vi "optimized_eod_recorder.vi"() -> ()   [LabVIEW 2014]
uses:
  Dropbox (MSU Efish Lab)/Undergraduates/Sarah_Sam/To Github/eodrecorderstates.ctl
  <vilib>/_DAQmxBase/Internals/DAQmxBase Read (Analog 2D DBL NChan NSamp).vi
  <vilib>/_DAQmxBase/Internals/DAQmxBase Timing (Sample Clock).vi
  <vilib>/_DAQmxBase/Internals/DAQmxBase Create Channel (AI-Voltage-Basic).vi
  <vilib>/Utility/miscctls.llb/LVCursorListTypeDef.ctl
  <vilib>/Utility/error.llb/DialogType.ctl
panel:
  in  "stop":bool
  in  "index (row)":i32
  out "Tab Control 3":enum32{"Page 1", "Page 2"}(tab)
  out "Waveform Graph":waveform(dbl)(graph)
  in  "Graph Time Base (sec)":dbl=1.0 format="%#_13g"
  out "Threshold":sgl
  out "Threshold 2":sgl
  out "Waveform Graph 2":waveform(dbl)(graph)
  out "Channel Name":string
  in  "Stop":bool caption="stop"
  out "Pre-Trigger Error Indicator":bool caption="Error Indicator\n(Indicates if trigger occurs before\npre-trigger samples were acquired)"
  out "# Pretrigger Samples\nAcquired":i32
  in  "RightSideControls":T1={"Open Data"=FALSE, "Capture"=FALSE, "LiveDataMode"=FALSE, "Sample Rate  (Hz)"=10000.0, "Length (Sec)"=0.05}
  out "ModeDisplay":string
  in  "Device in":tag="Dev1"
  in  "Channel":tag="Dev1/ai0"
  out "Tab Control":enum32{"Live Data", "Edit Data", "View Data"}(tab)
  in  "Tab Control 2":enum32{"Enter Data", "View Data"}(tab)
  in  "RecordDataControls":T2
  in  "Path":path
  in  "Waveform_Data_Entry":T3={"Species"="", "Comments"="", "Recording Temp °C"="", "Locality Code"="", "Specimen No."="", "Date"="", "Time"="", "Coupling"=FALSE, "Polarity 2"=FALSE, "Gain"=10000.0} {"Gain" step=1.0 scale=1.0..50000.0 scale format="%#_6e"}
  out "EodText":string[](array[string])
  out "Polarity":i32[](array[numeric])
  out "Npts":i32[](array[numeric])
  out "Srate":i32[](array[numeric])
  out "ADRange":dbl[](array[numeric])
  in  "WaveNumber":i32(slide)=1 min=0 step=1 scale=1.0..3.0 scale format="%#.0f"
  # "EOD Recorder v. 1.0"
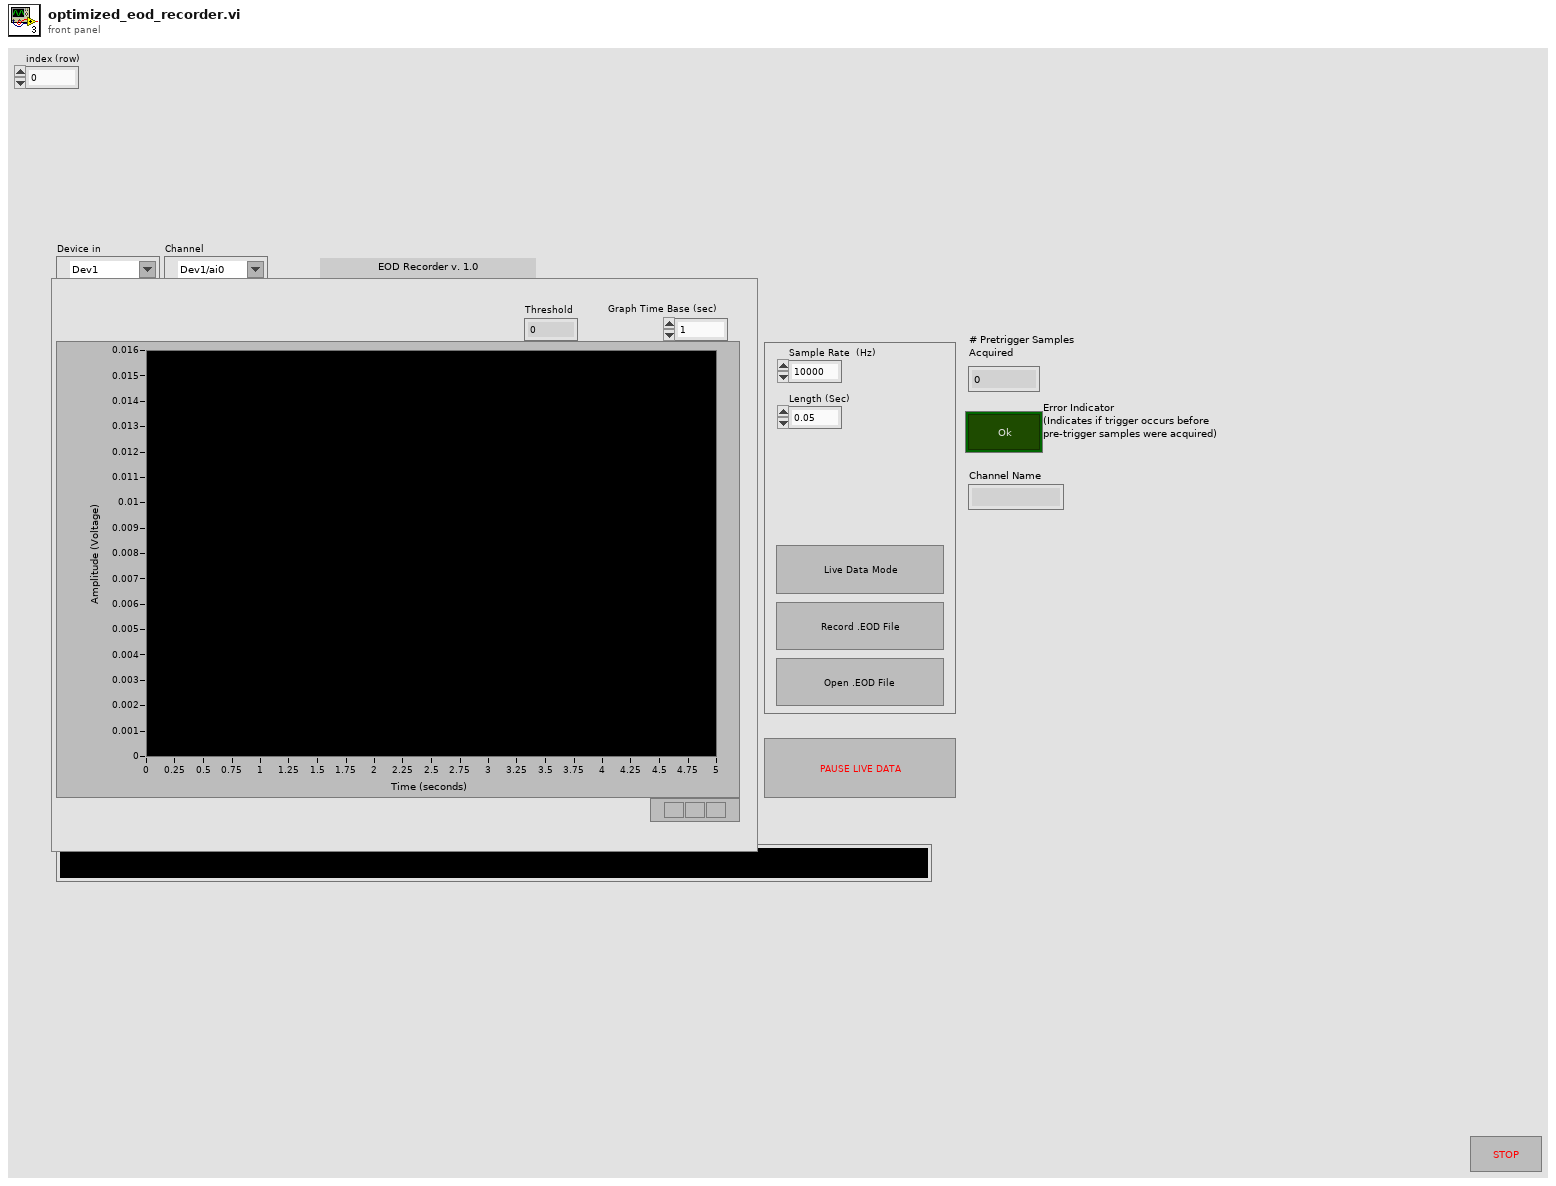
[diagram p1: front panel]
types:
  T1 = cluster{"Open Data":bool, "Capture":bool, "LiveDataMode":bool, "Sample Rate  (Hz)":dbl, "Length (Sec)":dbl}
  T2 = cluster{"Discard&Continue":bool, "Save&Finish":bool, "Save&Continue":bool, "StartOver":bool}
  T3 = cluster{"Species":string, "Comments":string, "Recording Temp °C":string, "Locality Code":string, "Specimen No.":string, "Date":string, "Time":string, "Coupling":bool, "Polarity 2":bool, "Gain":dbl}
  T4 = cluster{"Cursor.Cursor Y":dbl, "XScale.Maximum":dbl, "XScale.Minimum":dbl, "YScale.Maximum":dbl, "YScale.Minimum":dbl}
  T5 = typedef "eodrecorderstates.ctl" = enum16{"copy_scale_info", "setup", "stop", "initialize", "live data", "capture data", "analyze data", "pause live data", "open data", "display opened data", "view_collected_data", "write to file", "audio_live"}
  T6 = cluster{"data":dbl[][], "task ":refnum<k21>, "error ":errorcluster, "Min":dbl, "Max":dbl, "LastGrabbedSrate":dbl, "OpenedWaveformData":cluster{"Nchar":i32[], "EodText":string[], "Nbits":i32[], "Nbytes":i32[], "userdata":dbl[][], "Polarity":i32[], "Srate":i32[], "ADRange":dbl[], "Npts":i32[], "Wave":dbl[][]}, "NumberofWavesLoaded":i32, "lastgrabbedsamples":i32, "LastCapturedWaveformData":cluster{"Nchar":i32, "EodText":string, "Nbits":i32, "Nbytes":i32, "userdata":dbl, "Polarity":i32, "Srate":i32, "Npts":i32, "Wave":waveform(dbl), "Version":i32}}
  T7 = typedef "LVCursorListTypeDef.ctl" = cluster{"Name":string, "Color":u32, "Style":u8, "Point Style":u8, "Name Visible":bool, "Allow Drag":bool, "Cursor Mode":u32, "Plot":i32, "Index":i32, "Position":cluster{"X":dbl, "Y":dbl}, "X Scale":u32, "Y Scale":u32, "Watch Plots":i32[], "Watch All Plots":bool, "Plot Area":i32, "Label Offset":cluster{"X":dbl, "Y":dbl}}[]
  T8 = enum16{"Rising Edge", "Falling Edge", "Above Level", "Below Level", "When Inside Window", "When Outside Window"}
  T9 = enum16{"open", "replace", "create", "open or create", "replace or create", "replace or create with confirmation"}
  T10 = typedef "DialogType.ctl" = u16
  T11 = cluster{"Nchar":i32[], "EodText":string[], "Nbits":i32[], "Nbytes":i32[], "userdata":dbl[][], "Polarity":i32[], "Srate":i32[], "ADRange":dbl[], "Npts":i32[], "Wave":dbl[][]}
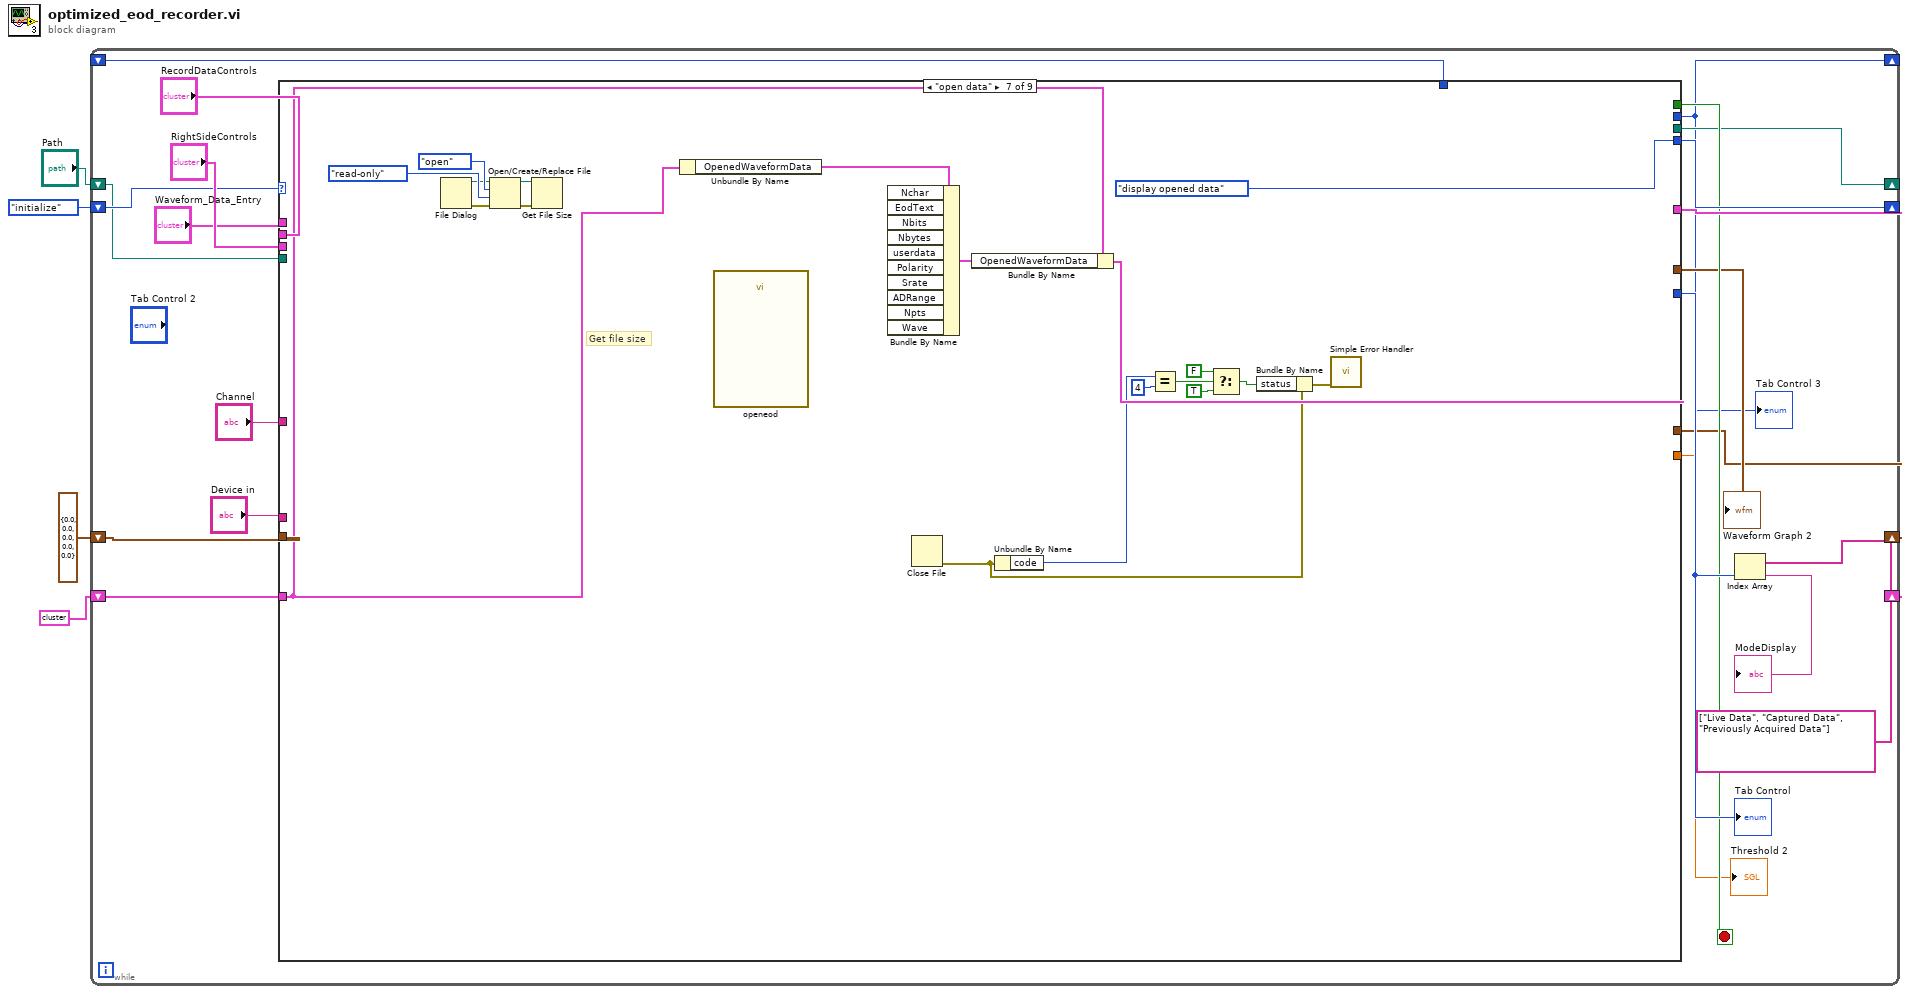
[diagram p0: block diagram]
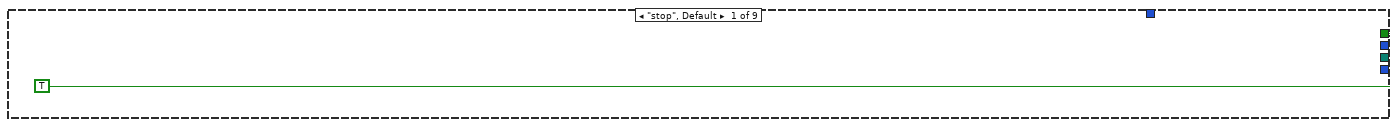
[diagram p2: hidden frame]
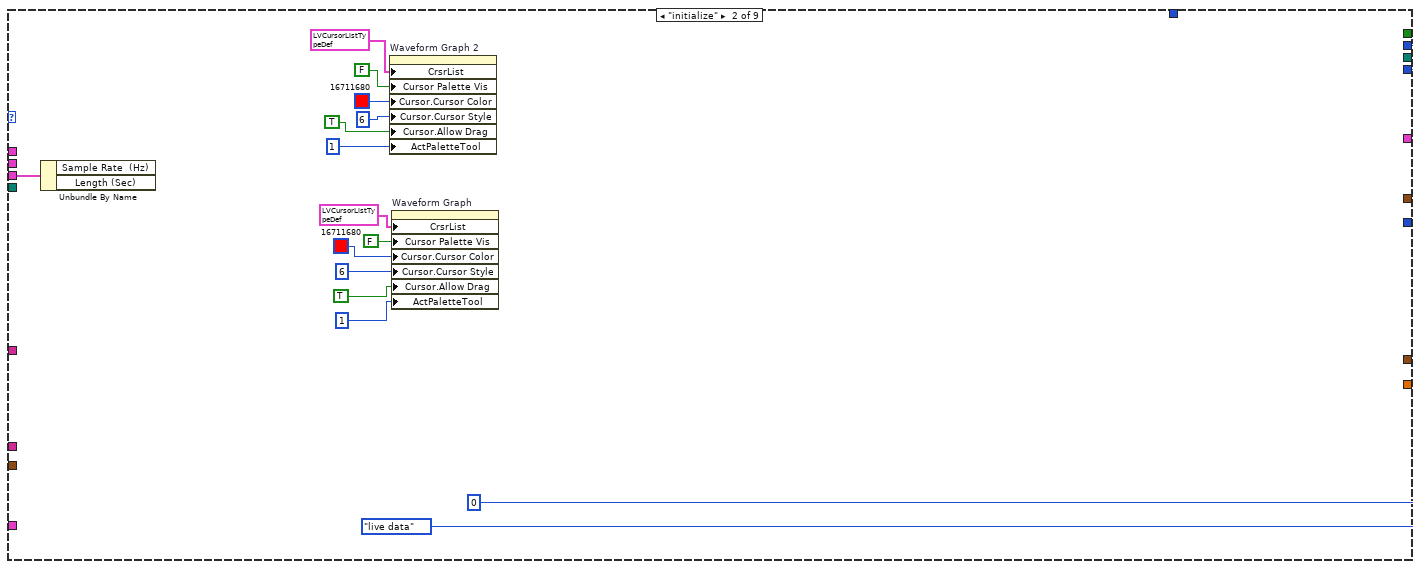
[diagram p3: hidden frame]
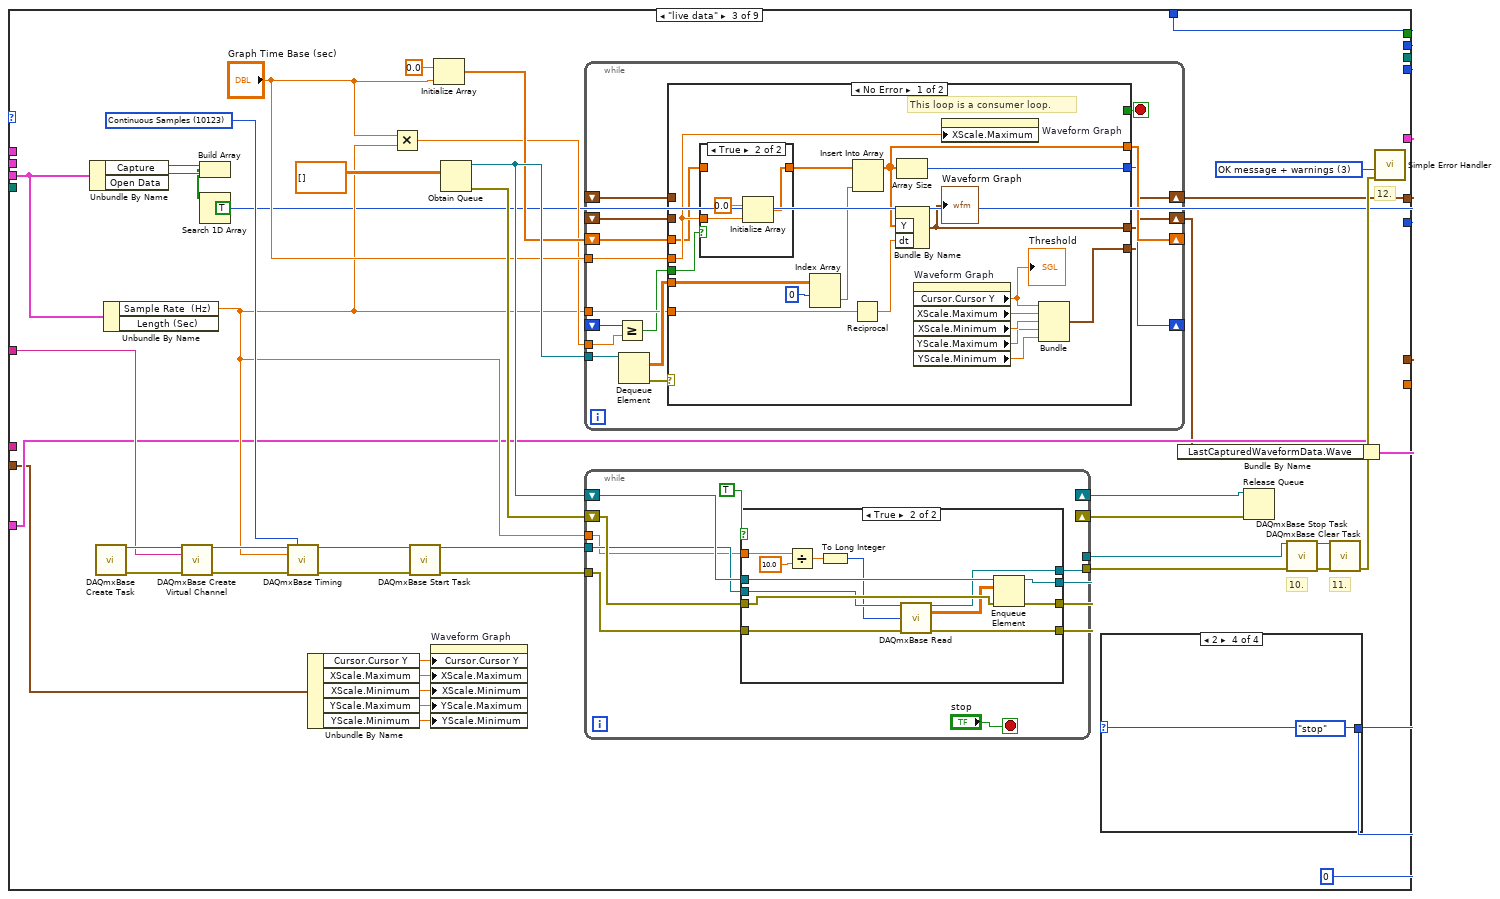
[diagram p4: hidden frame]
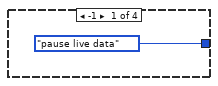
[diagram p5: hidden frame]
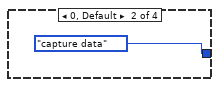
[diagram p6: hidden frame]
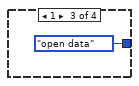
[diagram p7: hidden frame]
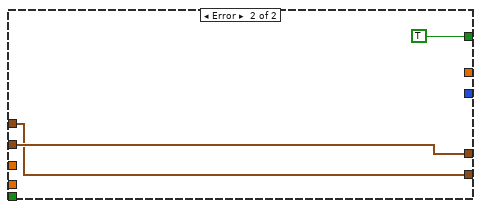
[diagram p9: hidden frame]
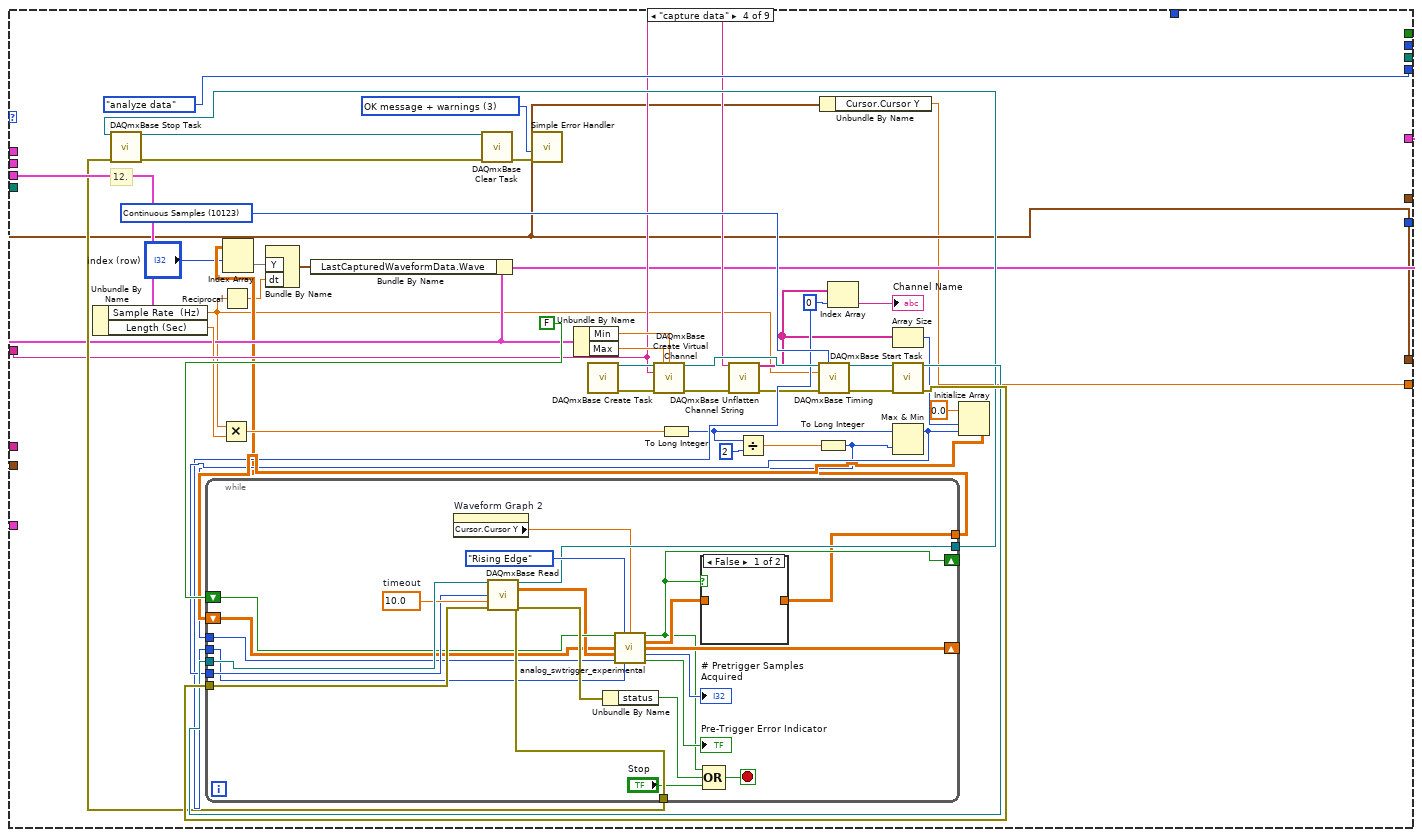
[diagram p11: hidden frame]
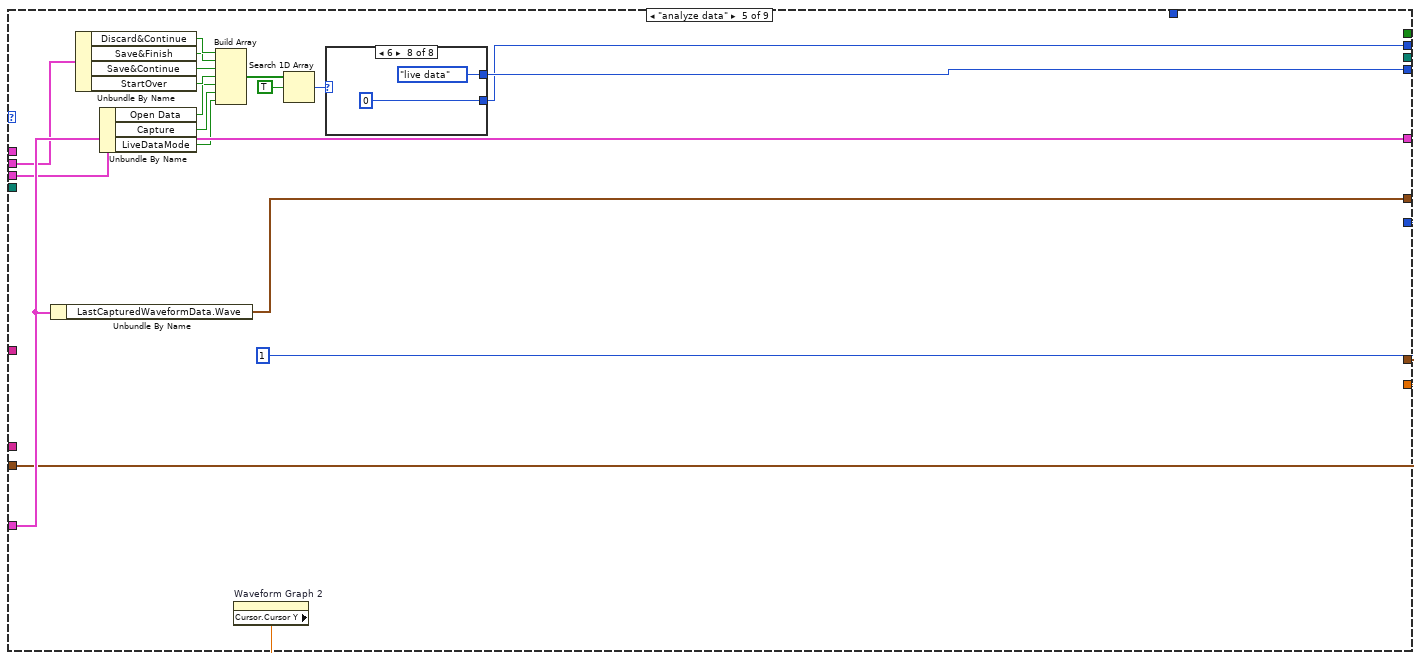
[diagram p13: hidden frame]
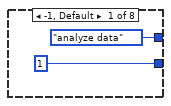
[diagram p14: hidden frame]
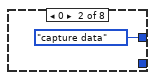
[diagram p15: hidden frame]
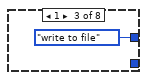
[diagram p16: hidden frame]
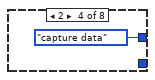
[diagram p17: hidden frame]
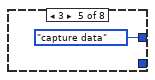
[diagram p18: hidden frame]
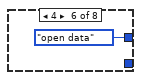
[diagram p19: hidden frame]
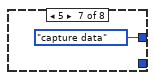
[diagram p20: hidden frame]
diagram:
  n1 = while {
    shift-right: [w21] -> _
    shift-left: T6 {"data"=[], "task "="", "error "={"status"=FALSE, "code"=0, "source"=""}, "Min"=-10.0, "Max"=10.0, "LastGrabbedSrate"=100000.0, "OpenedWaveformData"={"Nchar"=[], "EodText"=[], "Nbits"=[], "Nbytes"=[], "userdata"=[], "Polarity"=[], "Srate"=[], "ADRange"=[], "Npts"=[], "Wave"=[]}, "NumberofWavesLoaded"=4, "lastgrabbedsamples"=0, "LastCapturedWaveformData"={"Nchar"=0, "EodText"="", "Nbits"=0, "Nbytes"=0, "userdata"=0.0, "Polarity"=0, "Srate"=0, "Npts"=0, "Wave"={"t0"=timestamp(0 s since 1904-01-01), "dt"=1.0, "Y"=[]}, "Version"=0}} -> [w25]
    shift-right: [w20] -> _
    shift-left: eodrecorderstates."initialize" ("Enum") -> [w19]
    shift-right: [w12] -> _
    shift-left: "Path" -> [w13]
    shift-right: [w9] -> _
    shift-left: T4 {"Cursor.Cursor Y"=0.0, "XScale.Maximum"=0.0, "XScale.Minimum"=0.0, "YScale.Maximum"=0.0, "YScale.Minimum"=0.0} -> [w8]
    shift-right: [w6] -> _
    shift-left: _ -> [w5]
    stop <- w15 stop-if-true
    n2 = case shown="\"open data\"" w19 {
      tunnel: w25 -> [_ _ w51 w169 w246 w278 w291 w314 w343]
      tunnel: "Device in" -> [_ _ _ _ _ _ _ _ _]
      tunnel: "Channel" -> [_ _ w60 w176 _ _ _ _ _]
      tunnel: "RightSideControls" -> [_ w41 w86 w204 w234 w266 _ w305 _]
      tunnel: [_ _ w49 w168 w246 w278 w289 w314 _] -> w21
      tunnel: [_ eodrecorderstates."live data" ("Enum") w53 eodrecorderstates."analyze data" ("Enum") w237 eodrecorderstates."analyze data" ("Enum") eodrecorderstates."display opened data" ("Enum") w300 _] -> w20
      tunnel: [_ _ 0 _ 1 1 _ 2 _] -> w16
      tunnel: [TRUE _ _ _ _ _ _ _ _] -> w15
      tunnel: "Waveform_Data_Entry" -> [_ _ _ _ _ _ _ _ w351]
      tunnel: w13 -> [_ _ _ _ _ _ _ _ w337]
      tunnel: [_ _ _ _ _ _ _ _ w336] -> w12
      tunnel: "RecordDataControls" -> [_ _ _ _ w245 w277 _ _ _]
      tunnel: [_ _ _ _ w235 w267 _ _ _] -> w10
      tunnel: [_ 0 w42 _ w229 1 _ _ _] -> w6
      tunnel: [_ _ w52 w161 w228 w257 _ _ _] -> w9
      tunnel: w8 -> [_ _ w48 w161 w228 w257 _ _ _]
      tunnel: [_ _ _ w160 w230 _ _ _ _] -> w7
      tunnel: w5 -> [_ _ w42 _ _ _ _ _ _]
      frame "stop", Default {
      }
      frame "initialize" {
        n3 = Unbundle By Name(w41) -> ()  [unwired: 2 out]
        n4 = property on="Waveform Graph 2" class="WFGraph (strict)"("CrsrList"=T7 [{"Name"="Threshold\n", "Color"=0, "Style"=0, "Point Style"=0, "Name Visible"=FALSE, "Allow Drag"=TRUE, "Cursor Mode"=0, "Plot"=0, "Index"=0, "Position"={"X"=-inf, "Y"=0.0}, "X Scale"=0, "Y Scale"=0, "Watch Plots"=[], "Watch All Plots"=FALSE, "Plot Area"=0, "Label Offset"={"X"=0.0, "Y"=0.0}}] ("Cursor List"), "Cursor Palette Vis"=FALSE ("Cursor Legend Visible"), "Cursor.Cursor Color"=u32 16711680, "Cursor.Cursor Style"=u8 6, "Cursor.Allow Drag"=TRUE, "ActPaletteTool"=1 ("Palette:Active Tool")) -> ()  [unwired: 2 in, 2 out]
        n5 = property on="Waveform Graph" class="WFGraph (strict)"("CrsrList"=T7 [{"Name"="Threshold\n", "Color"=0, "Style"=0, "Point Style"=0, "Name Visible"=FALSE, "Allow Drag"=TRUE, "Cursor Mode"=0, "Plot"=0, "Index"=0, "Position"={"X"=-inf, "Y"=0.0}, "X Scale"=0, "Y Scale"=0, "Watch Plots"=[], "Watch All Plots"=FALSE, "Plot Area"=0, "Label Offset"={"X"=0.0, "Y"=0.0}}] ("Cursor List"), "Cursor Palette Vis"=FALSE ("Cursor Legend Visible"), "Cursor.Cursor Color"=u32 16711680, "Cursor.Cursor Style"=u8 6, "Cursor.Allow Drag"=TRUE, "ActPaletteTool"=1 ("Palette:Active Tool")) -> ()  [unwired: 2 in, 2 out]
      }
      frame "live data" {
        w66 = T10 3 items=["no dialog", "OK message", "continue or stop message", "OK message + warnings", "continue/stop + warnings"] ("type of dialog (OK msg:1)")
        w72 = 10123 items=["Finite Samples"=10178, "Continuous Samples"=10123, "Hardware Timed Single Point"=12522] ("sample mode")
        # "12."
        # "11."
        # "10."
        n6 = Unbundle By Name(w86) -> ("Capture"=w58:bool, "Open Data"=w57:bool)
        n7 = call <vilib>:"DAQmxBase Create Task.vi"() -> ("task out"=w80:refnum<k21>, "error out"=w79:errorcluster)  [unwired: 5 in, 9 out]
        n8 = Unbundle By Name(w86) -> ("Sample Rate  (Hz)"=w59:dbl)  [unwired: 1 out]
        n9 = call-poly <vilib>:"DAQmxBase Create Virtual Channel.vi"("task in"=w80, "physical channels"=w60, "error in"=w79) -> ("task out"=w78:refnum<k21>, "error out"=w77:errorcluster)  [unwired: 6 in, 5 out]
        n10 = Build Array(w58, w57) -> (w56:bool[])
        n11 = Search 1D Array(1D array=w56, element=TRUE) -> (index of element=w54:i32)  [unwired: 1 in]
        n12 = call-poly <vilib>:"DAQmxBase Timing.vi"("task/channels in"=w78, "sample mode"=w72, "rate"=w59, "error in"=w77) -> ("task out"=w76:refnum<k21>, "error out"=w75:errorcluster)  [unwired: 3 in, 7 out]
        n13 = Unbundle By Name(w48) -> ("Cursor.Cursor Y"=w47:dbl, "XScale.Maximum"=w46:dbl, "XScale.Minimum"=w45:dbl, "YScale.Maximum"=w44:dbl, "YScale.Minimum"=w43:dbl)
        n14 = Multiply(x="Graph Time Base (sec)", y=w59) -> (x*y=w61:dbl)
        n15 = call <vilib>:"DAQmxBase Start Task.vi"("task/channels in"=w76, "error in"=w75) -> ("task out"=w74:refnum<k21>, "error out"=w73:errorcluster)  [unwired: 12 out]
        n16 = property on="Waveform Graph" class="WFGraph (strict)"("Cursor.Cursor Y"=w47, "XScale.Maximum"=w46, "XScale.Minimum"=w45, "YScale.Maximum"=w44, "YScale.Minimum"=w43) -> ()  [unwired: 2 in, 2 out]
        n17 = Initialize Array(0.0 ("element"), "Graph Time Base (sec)") -> (w63:dbl[])
        n18 = Obtain Queue(element data type=dbl[][] [] ("data")) -> (queue out=w84:refnum<queue>, error out=w83:errorcluster)  [unwired: 4 in, 1 out]
        n19 = while {
          tunnel: w84 -> [w106]
          tunnel: w59 -> [w102]
          tunnel: "Graph Time Base (sec)" -> [w101]
          shift-right: [w99] -> _
          shift-left: w63 -> [w100]
          shift-right: [w98] -> _
          shift-left: _ -> [w97]
          tunnel: w61 -> [w95]
          shift-right: [w94] -> w50
          shift-left: _ -> [w92]
          shift-right: [w93] -> w52
          shift-left: _ -> [w91]
          stop <- w103 stop-if-true
          # "This loop is a consumer loop."
          n20 = Greater Or Equal?(x=w97, y=w95) -> (x >= y?=w96:bool)
          n21 = Dequeue Element(queue=w106) -> (element=w104:dbl[][], error out=w105:errorcluster)  [unwired: 2 in, 2 out]
          n22 = case shown="No Error" w105 {
            tunnel: w104 -> [w124 _]
            tunnel: [_ TRUE] -> w103
            tunnel: w102 -> [w121 _]
            tunnel: w101 -> [w116 _]
            tunnel: [w119 _] -> w99
            tunnel: w100 -> [w115 _]
            tunnel: [w118 _] -> w98
            tunnel: w96 -> [w117 _]
            tunnel: [w113 w130] -> w94
            tunnel: [w108 w129] -> w93
            tunnel: w92 -> [_ w130]
            tunnel: w91 -> [_ w129]
            frame No Error {
              n23 = case shown="True" w117 {
                tunnel: w116 -> [_ w127]
                tunnel: [w125 w126] -> w114
                tunnel: w115 -> [w125 _]
                frame False {
                }
                frame True {
                  n24 = Initialize Array(0.0 ("element"), w127) -> (w126:dbl[])
                }
              }
              n25 = Index Array(array=w124, index (row)=0) -> (element=w120:dbl[])  [unwired: 1 in]
              n26 = Reciprocal(x=w121) -> (1/x=w122:dbl)
              n27 = Insert Into Array(array=w114, new element=w120) -> (w119:dbl[])  [unwired: 1 in]
              n28 = Bundle By Name("Y"=w119, "dt"=w122) -> (w113:waveform(dbl))  [unwired: 1 in]
              "Waveform Graph" <- w113
              n29 = Array Size(array=w119) -> (size(s)=w118:i32)
              n30 = property on="Waveform Graph" class="WFGraph (strict)"() -> ("Cursor.Cursor Y"=w107:dbl, "XScale.Maximum"=w112:dbl, "XScale.Minimum"=w111:dbl, "YScale.Maximum"=w110:dbl, "YScale.Minimum"=w109:dbl)  [unwired: 2 in, 2 out]
              "Threshold" <- w107
              n31 = property on="Waveform Graph" class="WFGraph (strict)"("XScale.Maximum"=w116) -> ()  [unwired: 2 in, 2 out]
              n32 = Bundle("Cursor.Cursor Y"=w107, "XScale.Maximum"=w112, "XScale.Minimum"=w111, "YScale.Maximum"=w110, "YScale.Minimum"=w109) -> (w108:T4)  [unwired: 1 in]
            }
            frame Error {
            }
          }
        }
        n33 = while {
          shift-right: [w138] -> w81
          shift-left: w83 -> [w139]
          shift-right: [w140] -> w82
          shift-left: w84 -> [w141]
          tunnel: w74 -> [w136]
          tunnel: w73 -> [w135]
          tunnel: [w134] -> w68
          tunnel: [w133] -> w67
          tunnel: w59 -> [w132]
          stop <- "stop" stop-if-true
          n34 = case shown="True" TRUE ("Case Constant\n(See Context Help)") {
            tunnel: w141 -> [w146 w159]
            tunnel: [w146 w158] -> w140
            tunnel: w139 -> [w145 w157]
            tunnel: [w145 w156] -> w138
            tunnel: w136 -> [w143 w155]
            tunnel: w135 -> [w144 w154]
            tunnel: [w143 w153] -> w134
            tunnel: [w144 w152] -> w133
            tunnel: w132 -> [_ w150]
            frame False {
            }
            frame True {
              n35 = Divide(x=w150, y=10.0) -> (x/y=w147:dbl)
              n36 = To Long Integer(number=w147) -> (32bit integer=w148:i32)
              n37 = call-poly <vilib>:"DAQmxBase Read.vi"("task/channels in"=w155, "number of samples per channel"=w148, "error in"=w154) -> ("task out"=w153:refnum<k21>, "data"=w151:dbl[][], "error out"=w152:errorcluster)  [unwired: 1 in, 9 out]
              n38 = Enqueue Element(queue=w159, element=w151, error in (no error)=w157) -> (queue out=w158:refnum<queue>, error out=w156:errorcluster)  [unwired: 1 in, 1 out]
            }
          }
        }
        n39 = case shown="2" w54 {
          tunnel: [eodrecorderstates."pause live data" ("Enum") eodrecorderstates."capture data" ("Enum") eodrecorderstates."open data" ("Enum") eodrecorderstates."stop" ("Enum")] -> w53
          frame -1 {
          }
          frame 0, Default {
          }
          frame 1 {
          }
          frame 2 {
          }
        }
        n40 = Bundle By Name(cluster=w51, "LastCapturedWaveformData.Wave"=w50) -> (w49:T6)
        n41 = Release Queue(queue=w82, error in (no error)=w81) -> ()  [unwired: 1 in, 3 out]
        n42 = call <vilib>:"DAQmxBase Stop Task.vi"("task/channels in"=w68, "error in"=w67) -> ("task out"=w70:refnum<k21>, "error out"=w71:errorcluster)  [unwired: 12 out]
        n43 = call <vilib>:"DAQmxBase Clear Task.vi"("task in"=w70, "error in"=w71) -> ("error out"=w69:errorcluster)  [unwired: 13 out]
        n44 = call <vilib>:"Simple Error Handler.vi"("type of dialog (OK msg:1)"=w66, "error in (no error)"=w69) -> ()  [unwired: 8 out]
      }
      frame "capture data" {
        w190 = 0 ("Channel Index")
        w198 = T10 3 items=["no dialog", "OK message", "continue or stop message", "OK message + warnings", "continue/stop + warnings"] ("type of dialog (OK msg:1)")
        w199 = 10123 items=["Finite Samples"=10178, "Continuous Samples"=10123] ("sample mode")
        # "12."
        n45 = Unbundle By Name(w204) -> ("Sample Rate  (Hz)"=w163:dbl, "Length (Sec)"=w175:dbl)
        n46 = Multiply(x=w163, y=w175) -> (x*y=w174:dbl)
        n47 = Reciprocal(x=w163) -> (1/x=w164:dbl)
        n48 = Unbundle By Name(w169) -> ("Min"=w178:dbl, "Max"=w177:dbl)
        n49 = call <vilib>:"DAQmxBase Create Task.vi"() -> ("task out"=w183:refnum<k21>, "error out"=w184:errorcluster)  [unwired: 14 in]
        n50 = call-poly <vilib>:"DAQmxBase Create Virtual Channel.vi"("task in"=w183, "maximum value"=w177, "minimum value"=w178, "physical channels"=w176, "error in"=w184) -> ("task out"=w194:refnum<k21>, "error out"=w187:errorcluster)  [unwired: 9 in]
        n51 = To Long Integer(number=w174) -> (32bit integer=w173:i32)
        n52 = call "DAQmxBase Unflatten Channel String.vi"("names in"=w176, "error in"=w187) -> ("names out"=w186:string[], "error out"=w185:errorcluster)  [unwired: 12 in]
        n53 = Divide(x=w173, y=2) -> (x/y=w171:dbl)
        n54 = To Long Integer(number=w171) -> (32bit integer=w170:i32)
        n55 = call-poly <vilib>:"DAQmxBase Timing.vi"("task/channels in"=w194, "sample mode"=w199, "rate"=w163, "error in"=w185) -> ("task out"=w191:refnum<k21>, "error out"=w192:errorcluster)  [unwired: 10 in]
        n56 = Unbundle By Name(w161) -> ("Cursor.Cursor Y"=w160:dbl)
        n57 = Index Array(array=w186, index=w190) -> (element=→"Channel Name":string)
        n58 = Array Size(array=w186) -> (size(s)=w188:i32)
        n59 = call <vilib>:"DAQmxBase Start Task.vi"("task/channels in"=w191, "error in"=w192) -> ("task out"=w200:refnum<k21>, "error out"=w202:errorcluster)  [unwired: 12 in]
        n60 = Max & Min(x=w173, y=w170) -> (max(x,y)=w195:i32)  [unwired: 1 out]
        n61 = Initialize Array(0.0, w188, w195) -> (w196:dbl[][])
        n62 = while {
          tunnel: w202 -> [w226]
          tunnel: [w225] -> w182
          tunnel: w200 -> [w224]
          tunnel: [w210] -> w181
          tunnel: w195 -> [w222]
          shift-right: [w208] -> _
          shift-left: FALSE ("stop") -> [w221]
          shift-right: [w213] -> _
          shift-left: w196 -> [w205]
          tunnel: w170 -> [w216]
          tunnel: w190 -> [w209]
          tunnel: [w206] -> w167
          stop <- w218 stop-if-true
          w223 = 10.0  # timeout
          n63 = property on="Waveform Graph 2" class="WFGraph (strict)"() -> ("Cursor.Cursor Y"=w207:dbl)  [unwired: 2 in, 2 out]
          n64 = call-poly <vilib>:"DAQmxBase Read.vi"("task/channels in"=w224, "number of samples per channel"=w222, "timeout"=w223, "error in"=w226) -> ("task out"=w210:refnum<k21>, "data"=w214:dbl[][], "error out"=w225:errorcluster)  [unwired: 9 in]
          n65 = Unbundle By Name(w225) -> ("status"=w219:bool)
          n66 = call "analog_swtrigger_experimental.vi"("Triggered?"=w221, "Condition"=T8."Rising Edge", "Level"=w207, "Initialized Data Array"=w205, "Input Raw Data"=w214, "Pretrigger Samples"=w216, "Index of Condition Channel"=w209) -> ("Trigger Out"=w208:bool, "Output Data (Scaled)"=w212:dbl[][], "Raw Data Out"=w213:dbl[][], "# Pretrigger Samples"=→"# Pretrigger Samples\nAcquired":i32, "Pre-Trigger Error"=→"Pre-Trigger Error Indicator":bool)  [unwired: 3 in, 1 out]
          n67 = case shown="False" w208 {
            tunnel: w212 -> [_ w227]
            tunnel: [_ w227] -> w206
            frame False {
            }
            frame True {
            }
          }
          n68 = Compound Arithmetic op=OR(w208, w219, "Stop") -> (w218:bool)
        }
        n69 = call <vilib>:"DAQmxBase Stop Task.vi"("task/channels in"=w181, "error in"=w182) -> ("task out"=w180:refnum<k21>, "error out"=w179:errorcluster)  [unwired: 12 in]
        n70 = Index Array(array=w167, index (row)="index (row)") -> (element=w165:dbl[])  [unwired: 1 in]
        n71 = Bundle By Name("Y"=w165, "dt"=w164) -> (w162:waveform(dbl))  [unwired: 1 in]
        n72 = Bundle By Name(cluster=w169, "LastCapturedWaveformData.Wave"=w162) -> (w168:T6)
        n73 = call <vilib>:"DAQmxBase Clear Task.vi"("task in"=w180, "error in"=w179) -> ("error out"=w201:errorcluster)  [unwired: 13 in]
        n74 = call <vilib>:"Simple Error Handler.vi"("type of dialog (OK msg:1)"=w198, "error in (no error)"=w201) -> ()  [unwired: 3 in, 5 out]
      }
      frame "analyze data" {
        n75 = Unbundle By Name(w246) -> ("LastCapturedWaveformData.Wave"=w235:waveform(dbl))
        n76 = Unbundle By Name(w245) -> ("Discard&Continue"=w243:bool, "Save&Finish"=w242:bool, "Save&Continue"=w241:bool, "StartOver"=w240:bool)
        n77 = Unbundle By Name(w234) -> ("Open Data"=w233:bool, "Capture"=w232:bool, "LiveDataMode"=w231:bool)
        n78 = Build Array(w243, w242, w241, w240, w233, w232, w231) -> (w244:bool[])
        n79 = property on="Waveform Graph 2" class="WFGraph (strict)"() -> ("Cursor.Cursor Y"=w230:dbl)  [unwired: 2 in, 2 out]
        n80 = Search 1D Array(1D array=w244, element=TRUE) -> (index of element=w238:i32)  [unwired: 1 in]
        n81 = case shown="6" w238 {
          tunnel: [eodrecorderstates."analyze data" ("Enum") eodrecorderstates."capture data" ("Enum") eodrecorderstates."write to file" ("Enum") eodrecorderstates."capture data" ("Enum") eodrecorderstates."capture data" ("Enum") eodrecorderstates."open data" ("Enum") eodrecorderstates."capture data" ("Enum") eodrecorderstates."live data" ("Enum")] -> w237
          tunnel: [1 _ _ _ _ _ _ 0] -> w229
          frame -1, Default {
          }
          frame 0 {
          }
          frame 1 {
          }
          frame 2 {
          }
          frame 3 {
          }
          frame 4 {
          }
          frame 5 {
          }
          frame 6 {
          }
        }
      }
      frame "pause live data" {
        n82 = Unbundle By Name(w278) -> ("LastCapturedWaveformData.Wave"=w267:waveform(dbl))
        n83 = Unbundle By Name(w266) -> ("Open Data"=w265:bool, "Capture"=w264:bool, "LiveDataMode"=w263:bool)
        n84 = Unbundle By Name(w277) -> ("Discard&Continue"=w275:bool, "Save&Finish"=w274:bool, "Save&Continue"=w273:bool, "StartOver"=w272:bool)
        n85 = Unbundle By Name(w257) -> ("Cursor.Cursor Y"=w262:dbl, "XScale.Maximum"=w261:dbl, "XScale.Minimum"=w260:dbl, "YScale.Maximum"=w259:dbl, "YScale.Minimum"=w258:dbl)
        n86 = Build Array(w275, w274, w273, w272, w265, w264, w263) -> (w276:bool[])
        n87 = property on="Waveform Graph 2" class="WFGraph (strict)"("Cursor.Cursor Y"=w262, "XScale.Maximum"=w261, "XScale.Minimum"=w260, "YScale.Maximum"=w259, "YScale.Minimum"=w258) -> ()  [unwired: 2 in, 2 out]
        n88 = Search 1D Array(1D array=w276, element=TRUE) -> ()  [unwired: 1 in, 1 out]
      }
      frame "open data" {
        # "Get file size"
        n89 = File Dialog() -> (0:w294:errorcluster, 3:w287:path)  [unwired: 7 in, 2 out]
        n90 = Open/Create/Replace File(file path (use dialog)=w287, error in=w294, operation (0:open)=T9."open", access (0:read/write)=enum16{"read/write", "read-only", "write-only"}."read-only") -> (refnum out=w297:refnum<file>, error out=w293:errorcluster)  [unwired: 2 in, 1 out]
        n91 = Get File Size(file=w297, error in=w293) -> ()  [unwired: 3 out]
        n92 = Unbundle By Name(w291) -> ("OpenedWaveformData"=w292:T11)
        n93 = call "openeod.vi"() -> ()  [unwired: 17 in, 3 out]
        n94 = Bundle By Name(cluster=w292) -> (w290:T11)  [unwired: 10 in]
        n95 = Close File() -> (error out=w280:errorcluster)  [unwired: 2 in, 1 out]
        n96 = Bundle By Name(cluster=w291, "OpenedWaveformData"=w290) -> (w289:T6)
        n97 = Unbundle By Name(w280) -> ("code"=w286:i32)
        n98 = Equal?(x=w286, y=4) -> (x = y?=w284:bool)
        n99 = Select(t=FALSE, s=w284, f=TRUE) -> (s? t:f=w281:bool)
        n100 = Bundle By Name(cluster=w280, "status"=w281) -> (w279:errorcluster)
        n101 = call <vilib>:"Simple Error Handler.vi"("error in (no error)"=w279) -> ()  [unwired: 4 in, 5 out]
      }
      frame "display opened data" {
        n102 = Unbundle By Name(w314) -> ("OpenedWaveformData"=w321:T11)
        n103 = Unbundle By Name(w305) -> ("Open Data"=w303:bool, "Capture"=w298:bool, "LiveDataMode"=w302:bool)
        n104 = property on="WaveNumber" class="Slide (strict)"("Scale.Increment"=1.0 ("Scale.Range:Increment")) -> ()  [unwired: 2 in, 2 out]
        n105 = property on="WaveNumber" class="Slide (strict)"("Scale.Minimum"=1) -> ()  [unwired: 2 in, 2 out]
        n106 = Unbundle By Name(w321) -> ("EodText"=→"EodText":string[], "Polarity"=→"Polarity":i32[], "Srate"=→"Srate":i32[], "ADRange"=→"ADRange":dbl[], "Npts"=→"Npts":i32[], "Wave"=w317:dbl[][])  [unwired: 4 out]
        n107 = Build Array(w303, w298, w302) -> (w304:bool[])
        n108 = Search 1D Array(1D array=w304, element=TRUE) -> (index of element=w301:i32)  [unwired: 1 in]
        n109 = Subtract(x="WaveNumber", y=1) -> (x-y=w307:i32)
        n110 = Index Array(array=w317, index (row)=w307) -> (element=w316:dbl[])  [unwired: 1 in]
        n111 = Build Array(w307) -> (w318:i32[])
        n112 = property on="ADRange" class="Arr (strict)"("Index Values"=w318) -> ()  [unwired: 2 in, 2 out]
        n113 = property on="Npts" class="Arr (strict)"("Index Values"=w318) -> ()  [unwired: 2 in, 2 out]
        n114 = property on="Polarity" class="Arr (strict)"("Index Values"=w318) -> ()  [unwired: 2 in, 2 out]
        n115 = property on="Srate" class="Arr (strict)"("Index Values"=w318) -> ()  [unwired: 2 in, 2 out]
        n116 = property on="EodText" class="Arr (strict)"("Index Values"=w318) -> ()  [unwired: 2 in, 2 out]
        n117 = Build Array(w316) -> ()  [unwired: 1 out]
        n118 = case shown="1" w301 {
          tunnel: [eodrecorderstates."display opened data" ("Enum") eodrecorderstates."stop" ("Enum") eodrecorderstates."initialize" ("Enum") eodrecorderstates."initialize" ("Enum")] -> w300
          frame 0, Default {
          }
          frame 1 {
          }
          frame 2 {
          }
          frame 3 {
          }
        }
      }
      frame "write to file" {
        n119 = Unbundle By Name(w343) -> ("LastCapturedWaveformData.Nbits"=w328:i32, "LastCapturedWaveformData.Nbytes"=w340:i32, "LastCapturedWaveformData.userdata"=w339:dbl, "LastCapturedWaveformData.Polarity"=w342:i32, "LastCapturedWaveformData.Srate"=w341:i32, "LastCapturedWaveformData.Wave"=w335:waveform(dbl), "LastCapturedWaveformData.Version"=w338:i32, "Min"=w333:dbl, "Max"=w332:dbl)
        n120 = Subtract(x=w333, y=w332) -> (x-y=w331:dbl)
        n121 = Unbundle By Name(w335) -> ("Y"=w334:dbl[])
        n122 = Divide(x=w334, y=w331) -> (x/y=w330:dbl[])
        n123 = Power Of 2(x=w328) -> (2^x=w329:dbl)
        n124 = Multiply(x=w330, y=w329) -> (x*y=w327:dbl[])
        n125 = Unbundle By Name(w351) -> ("Species"=w350:string, "Comments"=w349:string, "Recording Temp °C"=w348:string, "Locality Code"=w347:string, "Specimen No."=w346:string, "Date"=w345:string, "Time"=w344:string)
        n126 = To Word Integer(number=w327) -> (16bit integer=w326:i16[])
        n127 = call "writeeodfile.vi"("Time"=w344, "Date"=w345, "Path"=w337, "Specimen"=w346, "Location"=w347, "Species"=w350, "UserData"=w339, "WaveformData"=w326, "NBits"=w328, "Version"=w338, "NBytes"=w340, "Comments"=w349, "Temp"=w348, "Sample Rate"=w341, "Polarity"=w342) -> ("Path Out"=w336:path)  [unwired: 4 in]
      }
    }
    "Tab Control" <- w16
    "Waveform Graph 2" <- w10
    "Tab Control 3" <- w6
    "Threshold 2" <- w7
    n128 = Index Array(array=string[] ["Live Data", "Captured Data", "Previously Acquired Data"], index=w16) -> (element=→"ModeDisplay":string)
  }
